vi "Sender.vi"() -> ()   [LabVIEW 2020, in "Data Communication Transmitter.lvlib"]
doc: "Sender VI. Sends the data to the receiver based on the user's inputs."
uses:
  Data Communication Transmitter.lvlib
  Typedefs/Mode Cluster.ctl
  Typedefs/Communication_Mode.ctl
  Typedefs/Communication_Type.ctl
  Typedefs/Medium.ctl
  Typedefs/Data Cluster.ctl
  Typedefs/Sender_Data_Cluster.ctl
  Typedefs/Timing Data.ctl
  Typedefs/Queue Operation_Sender.ctl
  Typedefs/User_Event_Operation.ctl
  Receiver/Typedefs/User event Operations.ctl
  Typedefs/Message type data.ctl
  Classes/Communication/Communication.lvclass
  Typedefs/User_Event_STOP.ctl
  Receiver/Data Communication Receiver.lvlib
  Classes/Children/Intra-Application/Children/Without data/Without Data.lvclass
panel:
  in  "Create Clone":bool
  in  "DATA":T1
  out "error out":errorcluster
  in  "error in":errorcluster
  in  "STOP":bool
  in  "Send":bool
  out "Status indicators":T2
  in  "Medium":T3
  in  "Mode":T4
  # "SENDER"
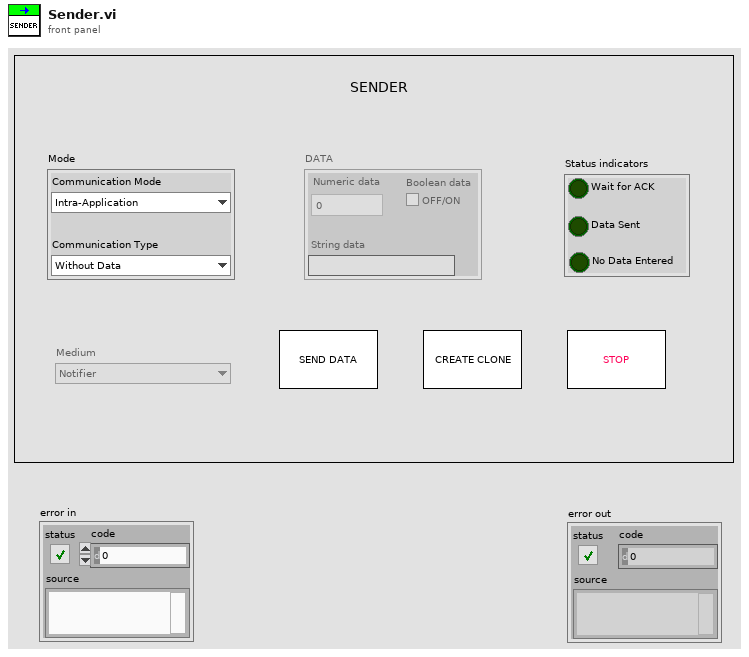
[diagram p1: front panel]
types:
  T1 = typedef "Data Communication Transmitter.lvlib/Data Cluster.ctl" = cluster{"Numeric data":dbl, "String data":string, "Boolean data":bool}
  T2 = cluster{"Wait for ACK":bool, "Data Sent":bool, "No Data Entered":bool}
  T3 = typedef "Data Communication Transmitter.lvlib/Medium.ctl" = enum16{"Notifier", "Queue"}
  T4 = typedef "Data Communication Transmitter.lvlib/Mode Cluster.ctl" = cluster{"Communication Mode":T5, "Communication Type":T6}
  T5 = typedef "Data Communication Transmitter.lvlib/Communication_Mode.ctl" = enum16{"Intra-Application", "Inter-Application"}
  T6 = typedef "Data Communication Transmitter.lvlib/Communication_Type.ctl" = enum16{"Without Data", "With Data"}
  T7 = typedef "Data Communication Transmitter.lvlib/User_Event_Operation.ctl" = enum16{"Create", "Generate", "Destroy", "Get Ref"}
  T8 = typedef "Data Communication Transmitter.lvlib/User event Operations.ctl" = enum16{"Create", "Generate", "Get Ref", "destroy"}
  T9 = typedef "Data Communication Transmitter.lvlib/Queue Operation_Sender.ctl" = enum16{"Create", "Enqueue", "Enstack", "Dequeue", "Flush", "Release"}
  T10 = typedef "Data Communication Transmitter.lvlib/Sender_Data_Cluster.ctl" = cluster{"Enable Controls ref":refnum<vi>[], "Disable Controls ref":refnum<vi>[], "File Path":path, "Status indicators":cluster{"Receiver Offline":bool, "Data Sent":bool, "No Data Entered":bool}, "Medium":T3, "DATA":T1, "Mode Cluster":T4, "Data type":string, "Timing":T11}
  T11 = typedef "Data Communication Transmitter.lvlib/Timing Data.ctl" = cluster{"Start Time":dbl, "Elapsed Time":dbl, "Previous Time":dbl, "Started?":bool, "Paused":bool, "Set Time":dbl}
  T12 = cluster{"Enable Controls ref":refnum<vi>[], "Disable Controls ref":refnum<vi>[]}
  T13 = cluster{"Receiver Offline":bool, "Data Sent":bool, "No Data Entered":bool}
  T14 = enum8{"Enabled", "Disabled", "Disabled and Grayed Out"}
  T15 = typedef "Data Communication Transmitter.lvlib/Message type data.ctl" = cluster{"Message type":string}
  T16 = cluster{"Numeric data":dbl, "String data":string, "Boolean data":bool}
  T17 = typedef "Data Communication Transmitter.lvlib/User_Event_STOP.ctl" = cluster{"STOP":bool}
  T18 = cluster{"Numeric data":bool, "String data":bool, "Boolean data":bool}
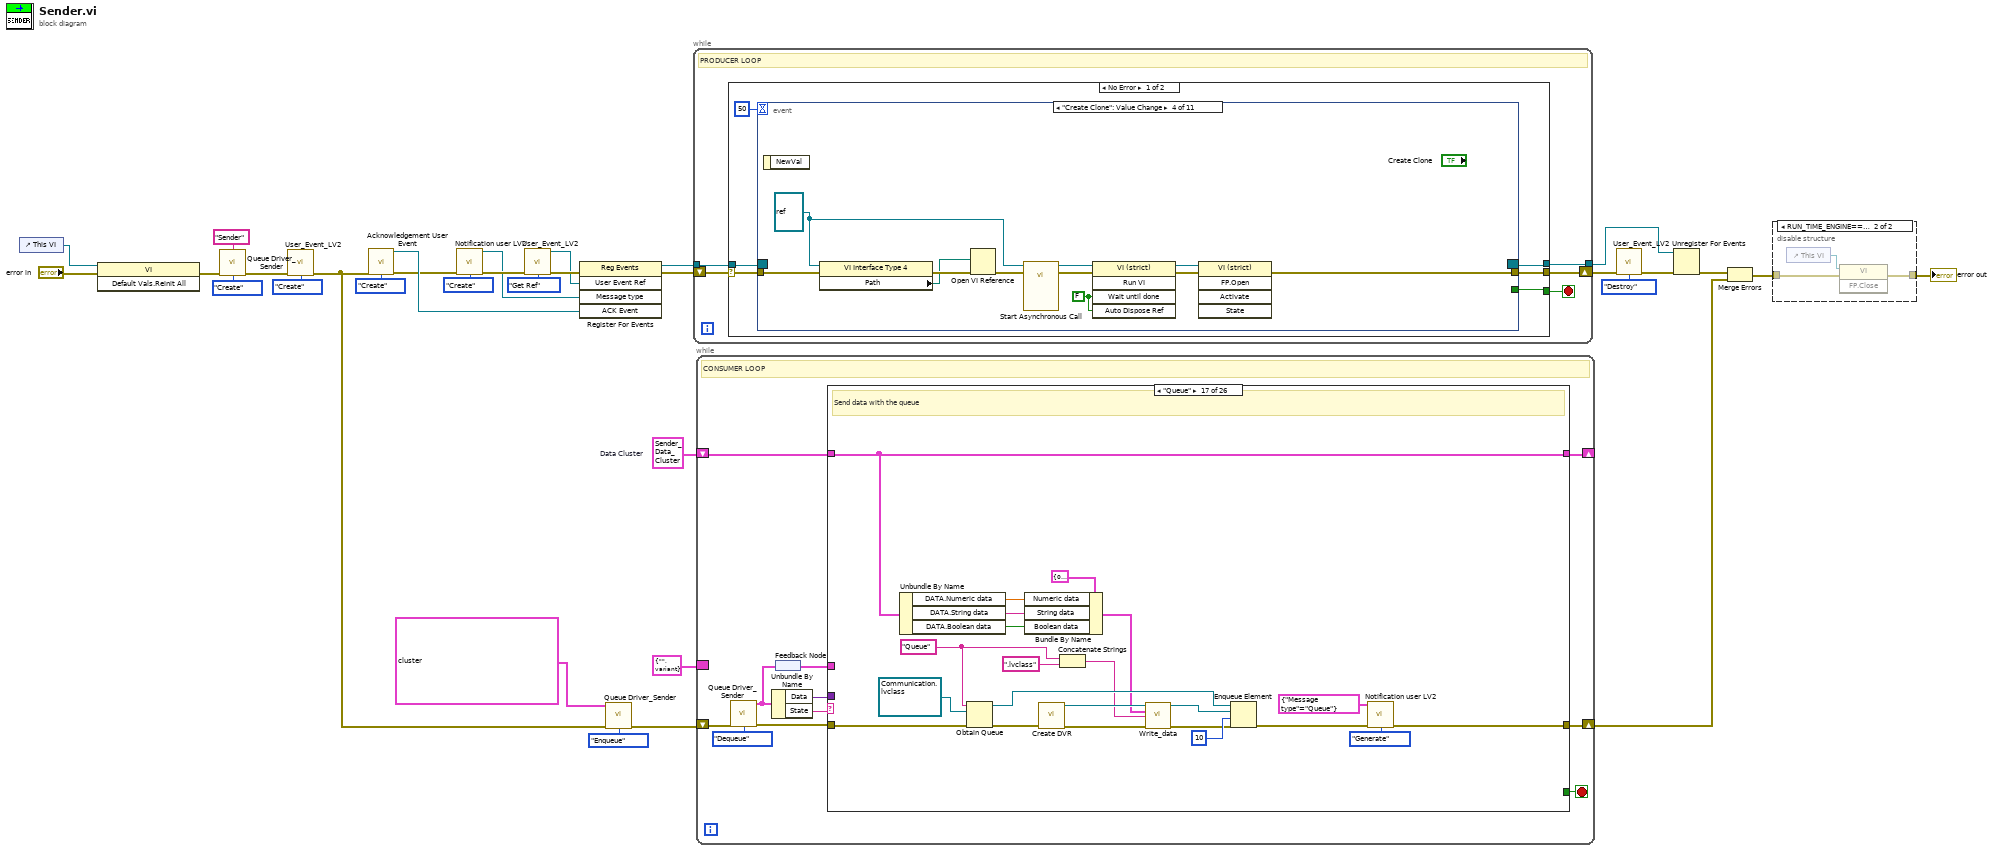
[diagram p0: block diagram]
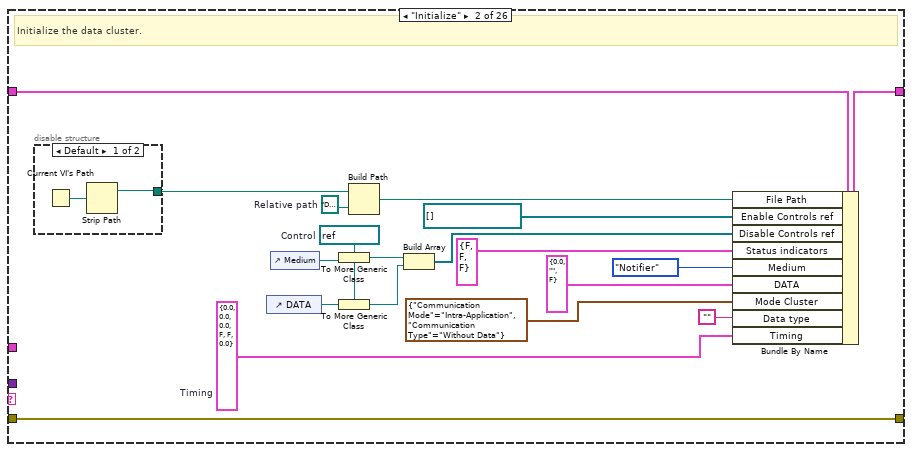
[diagram p4: hidden frame]
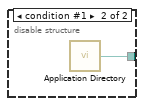
[diagram p5: hidden frame]
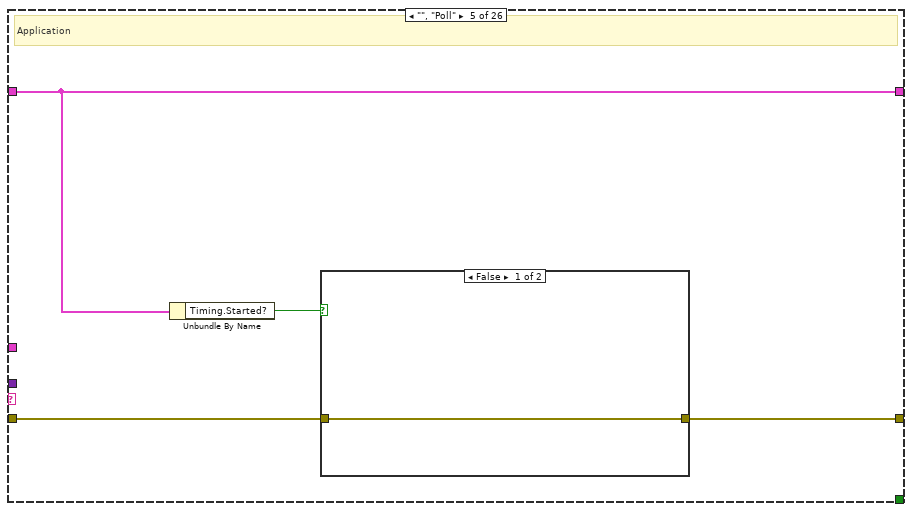
[diagram p8: hidden frame]
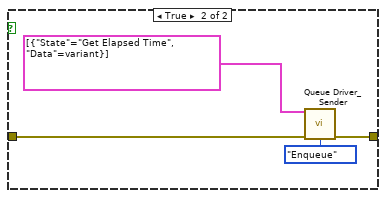
[diagram p9: hidden frame]
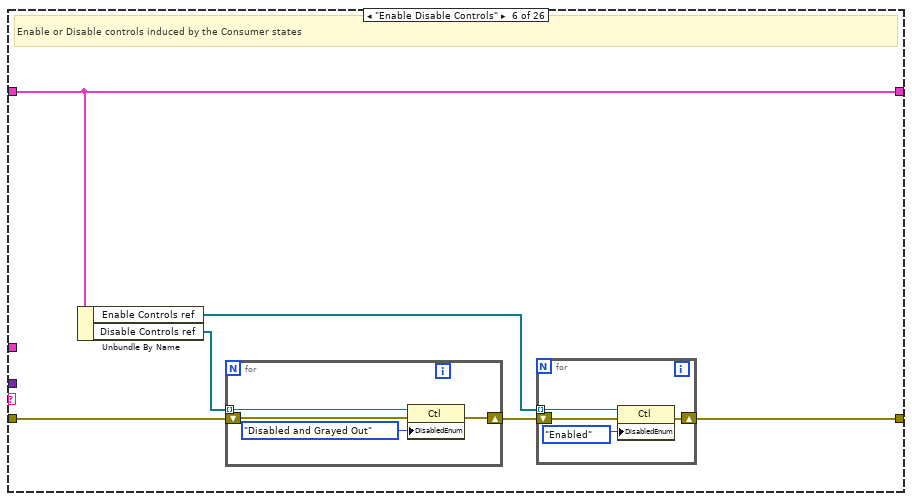
[diagram p10: hidden frame]
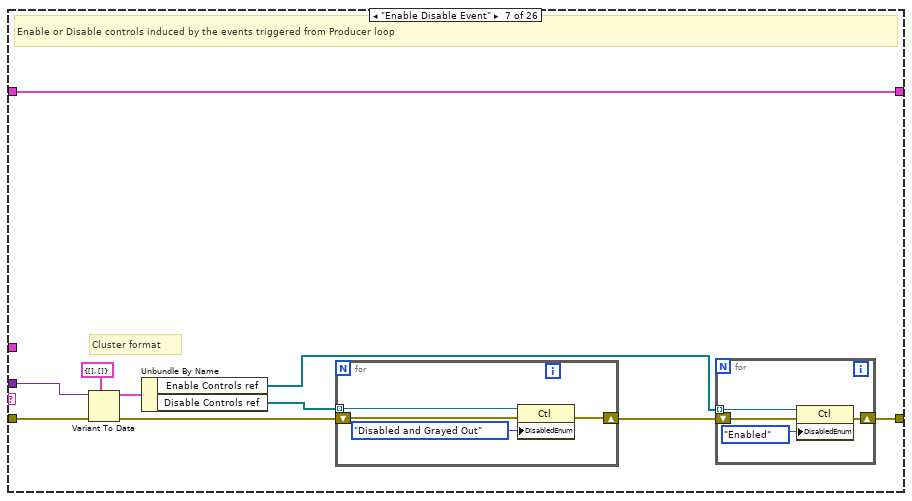
[diagram p11: hidden frame]
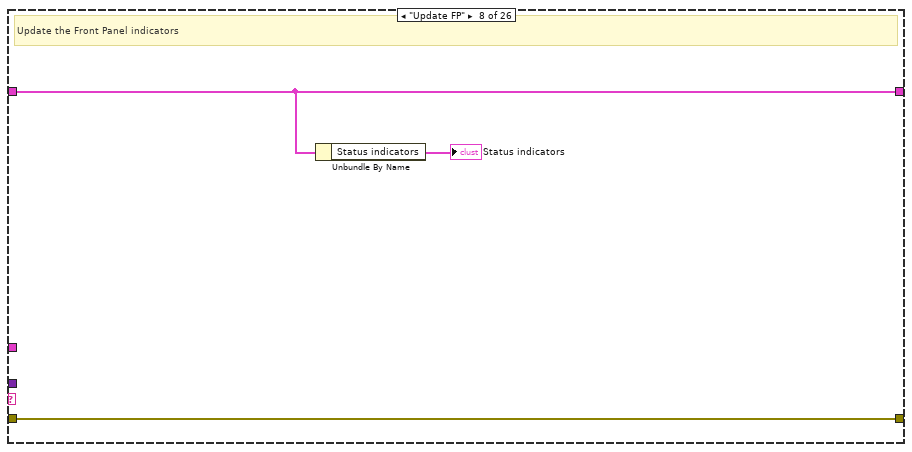
[diagram p12: hidden frame]
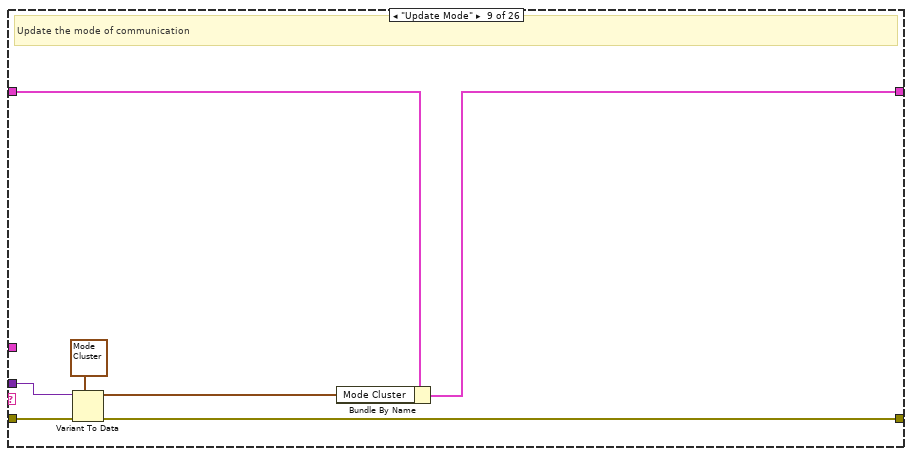
[diagram p13: hidden frame]
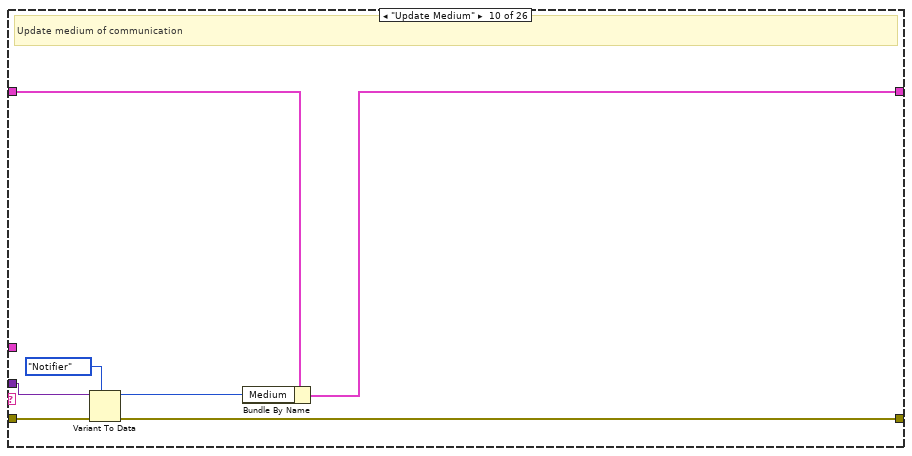
[diagram p14: hidden frame]
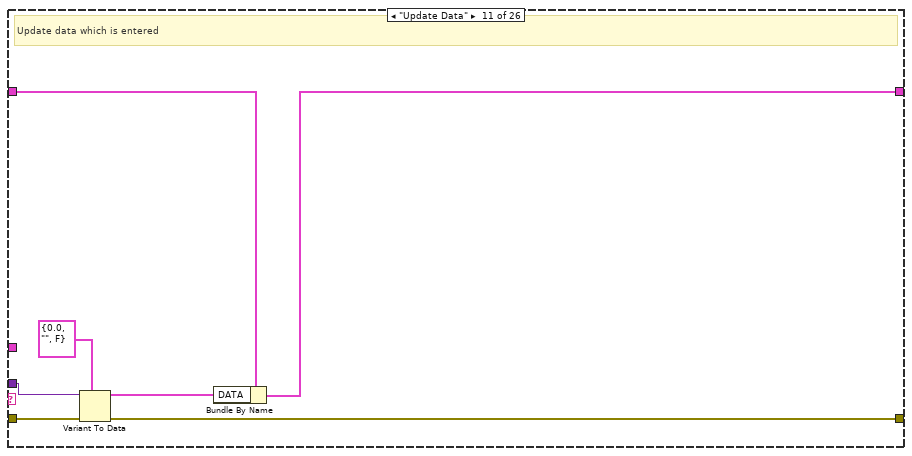
[diagram p15: hidden frame]
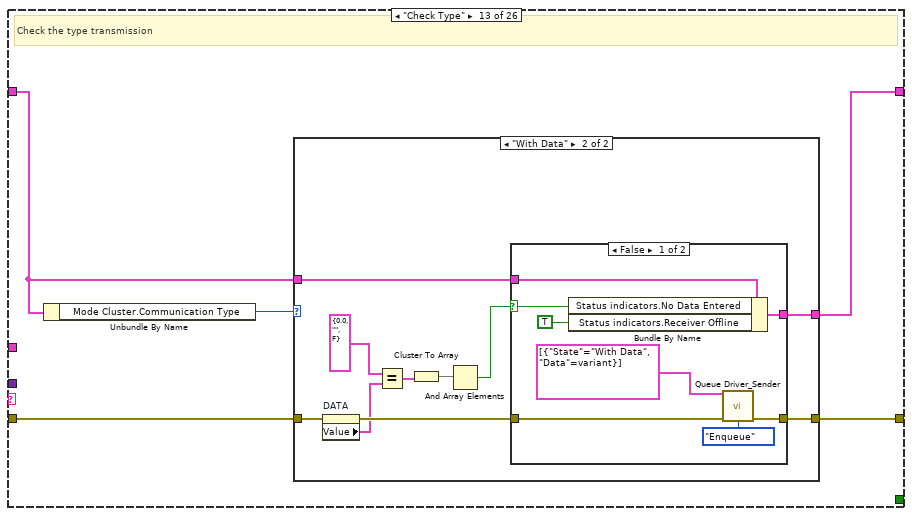
[diagram p17: hidden frame]
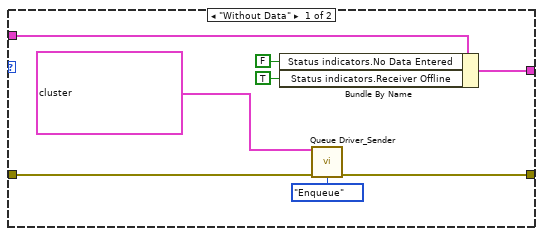
[diagram p18: hidden frame]
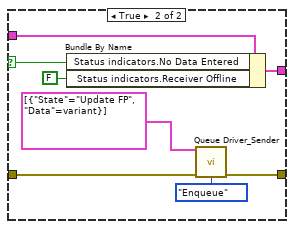
[diagram p19: hidden frame]
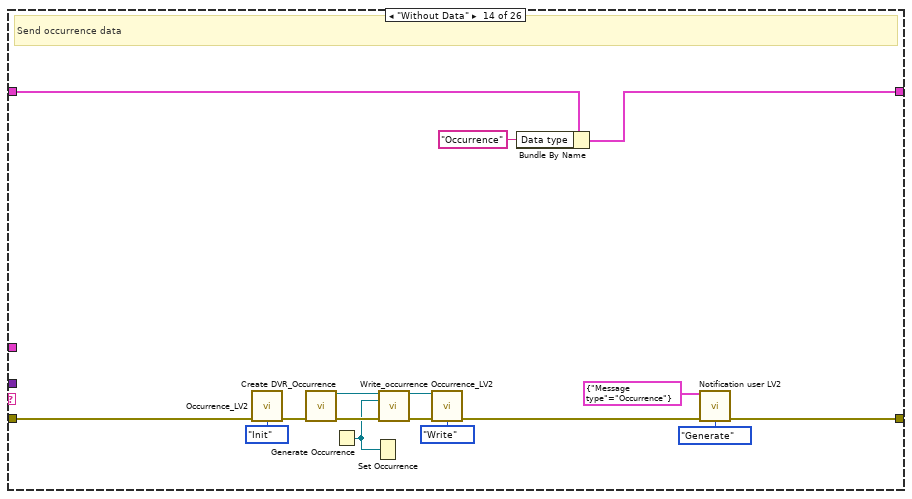
[diagram p20: hidden frame]
diagram:
  w32 = T10 {"Enable Controls ref"=[], "Disable Controls ref"=[], "File Path"=path "", "Status indicators"={"Receiver Offline"=FALSE, "Data Sent"=FALSE, "No Data Entered"=FALSE}, "Medium"=enum."Notifier", "DATA"={"Numeric data"=0.0, "String data"="", "Boolean data"=FALSE}, "Mode Cluster"={"Communication Mode"=enum."Intra-Application", "Communication Type"=enum."Without Data"}, "Data type"="", "Timing"={"Start Time"=0.0, "Elapsed Time"=0.0, "Previous Time"=0.0, "Started?"=FALSE, "Paused"=FALSE, "Set Time"=0.0}}  # Data Cluster
  n1 = control-ref of="This VI"() -> (w8:refnum<vi>)
  n2 = invoke on="Invoke Node" class="VI" method="Default Vals.Reinit All"(reference=w8, error in="error in") -> (error out=w10:errorcluster)  [unwired: 1 in, 2 out]
  n3 = call "Queue Driver_Sender.vi"("Queue Name"="Sender", "Error In"=w10, "Operation"=Queue_Operation_Sender."Create") -> ("Error Out"=w24:errorcluster)  [unwired: 11 in, 1 out]
  n4 = call "User_Event_LV2.vi"("Error In"=w24, "Operation"=User_Event_Operation."Create") -> ("Error Out"=w12:errorcluster)  [unwired: 12 in, 1 out]
  n5 = call "Acknowledgement User Event.vi"("Error in"=w12, "Operations"=User_event_Operations."Create") -> ("ACK Event"=w11:refnum<user-event>, "Error out"=w5:errorcluster)  [unwired: 12 in]
  n6 = call "Notification user LV2.vi"("Error In"=w5, "Operation"=User_Event_Operation."Create") -> ("Message type"=w3:refnum<user-event>, "Error Out"=w4:errorcluster)  [unwired: 12 in]
  n7 = call "User_Event_LV2.vi"("Error In"=w4, "Operation"=User_Event_Operation."Get Ref") -> ("User Event Ref"=w19:refnum<user-event>, "Error Out"=w21:errorcluster)  [unwired: 12 in]
  n8 = register-events(error in=w21, w19, w3, w11) -> (reference out=w18:refnum<event-registration>, error out=w20:errorcluster)  [unwired: 1 in]
  n9 = call "Queue Driver_Sender.vi"("Array of States"=cluster{"State":string, "Data":variant}[] [{"State"="Initialize", "Data"=variant}, {"State"="Enable Disable Controls", "Data"=variant}, {"State"="Update FP", "Data"=variant}], "Error In"=w12, "Operation"=Queue_Operation_Sender."Enqueue") -> ("Error Out"=w27:errorcluster)  [unwired: 11 in, 1 out]
  n10 = while {
    shift-right: [w36] -> w16
    shift-left: w20 -> [w37]
    tunnel: w18 -> [w35]
    tunnel: [w33] -> w13
    stop <- w34 stop-if-true
    # "PRODUCER LOOP"
    n11 = case shown="No Error" w37 {
      selector: w37 -> [w43 w158]
      tunnel: [w42 w164] -> w36
      tunnel: w35 -> [w41 w156]
      tunnel: [w40 _] -> w34
      tunnel: [w39 w156] -> w33
      frame No Error {
        n12 = event shown="[3] \"Create Clone\": Value Change" {
          selector: w41 -> [_ w46 _ _ _ _ _ _ _ _ _]
          dyn-events: [_ w46 _ _ _ _ _ _ _ _ _] -> w39
          timeout: 50 -> [_ _ _ _ _ _ _ _ _ _ _]
          tunnel: w43 -> [w45 w47 w52 w64 w71 w79 w89 w98 w107 w113 w118]
          tunnel: [w45 w47 w50 w55 w70 w78 w88 w103 w108 w114 w117] -> w42
          tunnel: [FALSE ("STOP") w48 FALSE ("STOP") _ FALSE ("STOP") FALSE ("STOP") FALSE ("STOP") FALSE ("STOP") FALSE ("STOP") FALSE ("STOP") FALSE ("STOP")] -> w40
          event Timeout {
            n13 = event-data() -> ()  [unwired: 1 in, 1 out]
          }
          event User Event {
            # "Consumer Stop Event"
            n14 = event-data() -> ("STOP"=w48:bool)  [unwired: 1 in]
          }
          event "Send": Value Change {
            # "Send Data"
            n15 = event-data() -> ()  [unwired: 1 in, 1 out]
            n16 = call "Queue Driver_Sender.vi"("Array of States"=cluster{"State":string, "Data":variant}[] [{"State"="Check Type", "Data"=variant}], "Error In"=w52, "Operation"=Queue_Operation_Sender."Enqueue") -> ("Error Out"=w50:errorcluster)  [unwired: 11 in, 1 out]
          }
          event "Create Clone": Value Change {
            w56 = FALSE ("Wait Until Done")
            w59 = refnum<vi> refnum
            n17 = event-data() -> ()  [unwired: 1 in, 1 out]
            n18 = property class="VI Interface Type 4"(reference=w59, error in=w64) -> (error out=w63:errorcluster, "Path"=w61:path)  [unwired: 1 out]
            n19 = Open VI Reference(vi path=w61, error in (no error)=w63) -> (error out=w62:errorcluster)  [unwired: 4 in, 1 out]
            n20 = call-by-ref "Start Asynchronous Call"(reference=w59, error in=w62) -> (reference out=w57:refnum<vi>, error out=w60:errorcluster)  [unwired: 15 in, 1 out]
            n21 = invoke class="VI (strict)" method="Run VI"(reference=w57, error in=w60, "Wait until done"=w56, "Auto Dispose Ref"=w56) -> (reference out=w54:refnum<vi>, error out=w58:errorcluster)  [unwired: 1 in, 3 out]
            n22 = invoke class="VI (strict)" method="FP.Open"(reference=w54, error in=w58) -> (error out=w55:errorcluster)  [unwired: 3 in, 4 out]
          }
          event Value Change {
            # "Update mode to cluster"
            n23 = event-data() -> ("NewVal"=w65:T4)  [unwired: 1 in]
            n24 = To Variant(anything=w65) -> (Variant=w66:variant)
            n25 = Bundle By Name(cluster=cluster{"State":string, "Data":variant} {"State"="", "Data"=variant} ("Data Cluster"), "State"="Update Mode", "Data"=w66) -> (w73:cluster{"State":string, "Data":variant})
            n26 = Build Array(w73) -> (w69:cluster{"State":string, "Data":variant}[])
            n27 = call "Queue Driver_Sender.vi"("Array of States"=w69, "Error In"=w71, "Operation"=Queue_Operation_Sender."Enqueue") -> ("Error Out"=w70:errorcluster)  [unwired: 11 in, 1 out]
          }
          event Value Change {
            # "Update medium of data transmission"
            n28 = event-data() -> ("NewVal"=w75:T3)  [unwired: 1 in]
            n29 = To Variant(anything=w75) -> (Variant=w76:variant)
            n30 = Bundle By Name(cluster=cluster{"State":string, "Data":variant} {"State"="", "Data"=variant} ("Data Cluster"), "State"="Update Medium", "Data"=w76) -> (w82:cluster{"State":string, "Data":variant})
            n31 = Build Array(w82) -> (w80:cluster{"State":string, "Data":variant}[])
            n32 = call "Queue Driver_Sender.vi"("Array of States"=w80, "Error In"=w79, "Operation"=Queue_Operation_Sender."Enqueue") -> ("Error Out"=w78:errorcluster)  [unwired: 11 in, 1 out]
          }
          event Value Change {
            # "Update change in input data"
            n33 = event-data() -> ("NewVal"=w85:T1)  [unwired: 1 in]
            n34 = To Variant(anything=w85) -> (Variant=w86:variant)
            n35 = Bundle By Name(cluster=cluster{"State":string, "Data":variant} {"State"="", "Data"=variant} ("Data Cluster"), "State"="Update Data", "Data"=w86) -> (w92:cluster{"State":string, "Data":variant})
            n36 = Build Array(w92) -> (w90:cluster{"State":string, "Data":variant}[])
            n37 = call "Queue Driver_Sender.vi"("Array of States"=w90, "Error In"=w89, "Operation"=Queue_Operation_Sender."Enqueue") -> ("Error Out"=w88:errorcluster)  [unwired: 11 in, 1 out]
          }
          event User Event {
            # "Acknowledgemnt from the receiver"
            n38 = event-data() -> ()  [unwired: 1 in, 1 out]
            n39 = property on="Data Sent" class="Bool (strict)"(error in=w98, "Value"=TRUE) -> (error out=w99:errorcluster)  [unwired: 1 in, 1 out]
            n40 = Bundle By Name(cluster=cluster{"State":string, "Data":variant} {"State"="", "Data"=variant} ("input cluster"), "State"="Start Timer") -> (w101:cluster{"State":string, "Data":variant})
            n41 = Build Array(w101) -> (w100:cluster{"State":string, "Data":variant}[])
            n42 = call "Queue Driver_Sender.vi"("Array of States"=w100, "Error In"=w99, "Operation"=Queue_Operation_Sender."Enqueue") -> ("Error Out"=w103:errorcluster)  [unwired: 11 in, 1 out]
          }
          event Panel Close? {
            # "Handling panel close"
            n43 = event-data() -> ()  [unwired: 1 in, 1 out]
            n44 = call "Queue Driver_Sender.vi"("Array of States"=cluster{"State":string, "Data":variant}[] [{"State"="Exit", "Data"=variant}], "Error In"=w107, "Operation"=Queue_Operation_Sender."Enqueue") -> ("Error Out"=w108:errorcluster)  [unwired: 11 in, 1 out]
            n45 = event-data ("Event Filter Node")("Discard?"=TRUE) -> ()  [unwired: 1 in, 1 out]
          }
          event "STOP": Value Change {
            # "Handle terminate with stop"
            n46 = event-data() -> ()  [unwired: 1 in, 1 out]
            n47 = call "Queue Driver_Sender.vi"("Array of States"=cluster{"State":string, "Data":variant}[] [{"State"="Exit", "Data"=variant}], "Error In"=w113, "Operation"=Queue_Operation_Sender."Enqueue") -> ("Error Out"=w114:errorcluster)  [unwired: 11 in, 1 out]
          }
          event Value Change {
            # "Enable and disbale controls"
            n48 = event-data() -> ("NewVal"=w119:T6)  [unwired: 1 in]
            n49 = case shown="\"Without Data\"" w119 {
              tunnel: w118 -> [w120 w138]
              tunnel: [w128 w147] -> w117
              frame "With Data" {
                w123 = refnum<vi> refnum  # Control
                n50 = control-ref of="DATA"() -> (w122:refnum<vi>)
                n51 = control-ref of="Medium"() -> (w136:refnum<vi>)
                n52 = To More Generic Class(target class=w123, reference=w136) -> (generic class reference=w135:refnum<vi>)
                n53 = To More Generic Class(target class=w123, reference=w122) -> (generic class reference=w121:refnum<vi>)
                n54 = Build Array(w135, w121) -> (w126:refnum<vi>[])
                n55 = Bundle By Name(cluster=T12 {"Enable Controls ref"=[], "Disable Controls ref"=[]} ("input cluster"), "Disable Controls ref"=refnum<vi>[] [], "Enable Controls ref"=w126) -> (w125:T12)
                n56 = To Variant(anything=w125) -> (Variant=w133:variant)
                n57 = Bundle By Name(cluster=cluster{"State":string, "Data":variant} {"State"="", "Data"=variant} ("Data Cluster"), "State"="Enable Disable Event", "Data"=w133) -> (w131:cluster{"State":string, "Data":variant})
                n58 = Build Array(w131) -> (w129:cluster{"State":string, "Data":variant}[])
                n59 = call "Queue Driver_Sender.vi"("Array of States"=w129, "Error In"=w120, "Operation"=Queue_Operation_Sender."Enqueue") -> ("Error Out"=w128:errorcluster)  [unwired: 11 in, 1 out]
              }
              frame "Without Data" {
                w142 = refnum<vi> refnum  # Control
                n60 = control-ref of="DATA"() -> (w141:refnum<vi>)
                n61 = control-ref of="Medium"() -> (w155:refnum<vi>)
                n62 = To More Generic Class(target class=w142, reference=w155) -> (generic class reference=w154:refnum<vi>)
                n63 = To More Generic Class(target class=w142, reference=w141) -> (generic class reference=w140:refnum<vi>)
                n64 = Build Array(w154, w140) -> (w145:refnum<vi>[])
                n65 = Bundle By Name(cluster=T12 {"Enable Controls ref"=[], "Disable Controls ref"=[]} ("input cluster"), "Enable Controls ref"=refnum<vi>[] [] ("Disable Controls ref"), "Disable Controls ref"=w145) -> (w144:T12)
                n66 = property on="No Data Entered" class="Bool (strict)"(error in=w138, "Value"=FALSE) -> (error out=w139:errorcluster)  [unwired: 1 in, 1 out]
                n67 = To Variant(anything=w144) -> (Variant=w152:variant)
                n68 = Bundle By Name(cluster=cluster{"State":string, "Data":variant} {"State"="", "Data"=variant} ("Data Cluster"), "State"="Enable Disable Event", "Data"=w152) -> (w150:cluster{"State":string, "Data":variant})
                n69 = Build Array(w150) -> (w148:cluster{"State":string, "Data":variant}[])
                n70 = call "Queue Driver_Sender.vi"("Array of States"=w148, "Error In"=w139, "Operation"=Queue_Operation_Sender."Enqueue") -> ("Error Out"=w147:errorcluster)  [unwired: 11 in, 1 out]
              }
            }
          }
        }
      }
      frame Error {
        n71 = To Variant(anything=w158) -> (Variant=w161:variant)
        n72 = call <vilib>:"Clear Errors.vi"("error in (no error)"=w158) -> ("error out"=w157:errorcluster)  [unwired: 5 in, 1 out]
        n73 = Bundle By Name(cluster=cluster{"State":string, "Data":variant} {"State"="", "Data"=variant} ("Data Cluster"), "State"="Producer Error", "Data"=w161) -> (w160:cluster{"State":string, "Data":variant})
        n74 = Build Array(w160) -> (w159:cluster{"State":string, "Data":variant}[])
        n75 = call "Queue Driver_Sender.vi"("Array of States"=w159, "Error In"=w157, "Operation"=Queue_Operation_Sender."Enqueue") -> ("Error Out"=w164:errorcluster)  [unwired: 11 in, 1 out]
      }
    }
  }
  n76 = while {
    shift-right: [w176] -> w26
    shift-left: w27 -> [w168]
    shift-right: [w172] -> _
    shift-left: w32 -> [w173]
    border: cluster{"State":string, "Data":variant} {"State"="", "Data"=variant} ("Data Cluster") -> [_]
    stop <- w174 stop-if-true
    # "CONSUMER LOOP"
    n77 = call "Queue Driver_Sender.vi"("Error In"=w168, "Operation"=Queue_Operation_Sender."Dequeue") -> ("Data Cluster"=w166:cluster{"State":string, "Data":variant}, "Error Out"=w169:errorcluster)  [unwired: 12 in]
    n78 = Unbundle By Name(w166) -> ("Data"=w175:variant, "State"=w171:string)
    n79 = feedback #1() -> (w170:cluster{"State":string, "Data":variant})
    n80 = feedback-in #1(w166) -> ()
    n81 = case shown="\"Queue\"" w171 {
      tunnel: [w178 w180 w202 w204 w206 w218 w235 w248 w249 w256 w266 w271 w274 w321 w329 w363 w381 w390 w393 w403 w412 w442 w445 w474 w493 w495] -> w176
      tunnel: w169 -> [w178 w180 w202 w204 w207 w215 w231 w248 w255 w262 w269 w271 w275 w320 w330 w358 w388 w390 w393 w403 w414 w442 w446 w471 w493 w498]
      tunnel: w175 -> [_ _ _ _ _ _ w230 _ w254 w261 w268 _ _ _ _ _ _ _ _ _ _ _ _ w473 _ _]
      tunnel: [_ _ _ _ _ _ _ _ _ _ _ _ _ _ _ _ _ _ _ _ _ _ _ _ _ TRUE] -> w174
      tunnel: w173 -> [w177 w194 w201 w203 w208 w214 w237 w247 w252 w259 w265 w270 w273 w326 w328 w366 w386 w389 w392 w402 w417 w441 w456 w481 w492 w503]
      tunnel: [w177 w193 w201 w203 w208 w214 w237 w247 w250 w258 w264 w270 w272 w325 w327 w366 w386 w389 w391 w401 w418 w441 w456 w481 w492 w503] -> w172
      tunnel: w170 -> [_ _ _ _ _ _ _ _ _ _ _ _ _ _ _ _ _ _ _ _ _ _ w444 _ _ _]
      frame "***Initialize***" {
      }
      frame "Initialize" {
        w181 = T11 {"Start Time"=0.0, "Elapsed Time"=0.0, "Previous Time"=0.0, "Started?"=FALSE, "Paused"=FALSE, "Set Time"=0.0}  # Timing
        w188 = refnum<vi> refnum  # Control
        w196 = path "Data/Accounts.csv"  # Relative path
        # "Initialize the data cluster."
        n82 = disable-structure "Conditional Disable Structure" shown="Default" {
          disable-tunnel: [w199 w200] -> w197
          frame condition #0 (active) {
            n83 = Current VI's Path() -> (path=w198:path)
            n84 = Strip Path(path=w198) -> (stripped path=w199:path)  [unwired: 1 out]
          }
          frame condition #1 {
            n85 = call <vilib>:"Application Directory.vi"() -> ("Application Directory"=w200:path)
          }
        }
        n86 = control-ref of="DATA"() -> (w187:refnum<vi>)
        n87 = control-ref of="Medium"() -> (w191:refnum<vi>)
        n88 = To More Generic Class(target class=w188, reference=w191) -> (generic class reference=w190:refnum<vi>)
        n89 = To More Generic Class(target class=w188, reference=w187) -> (generic class reference=w186:refnum<vi>)
        n90 = Build Path(base path=w197, name or relative path=w196) -> (appended path=w195:path)
        n91 = Build Array(w190, w186) -> (w189:refnum<vi>[])
        n92 = Bundle By Name(cluster=w194, "File Path"=w195, "Enable Controls ref"=refnum<vi>[] [], "Disable Controls ref"=w189, "Status indicators"=T13 {"Receiver Offline"=FALSE, "Data Sent"=FALSE, "No Data Entered"=FALSE}, "Medium"=Medium."Notifier", "DATA"=T1 {"Numeric data"=0.0, "String data"="", "Boolean data"=FALSE}, "Mode Cluster"=T4 {"Communication Mode"=enum."Intra-Application", "Communication Type"=enum."Without Data"}, "Data type"="" ("Empty String Constant"), "Timing"=w181) -> (w193:T10)
      }
      frame "***FP Related***" {
      }
      frame Default {
      }
      frame "", "Poll" {
        # "Application"
        n93 = Unbundle By Name(w208) -> ("Timing.Started?"=w205:bool)
        n94 = case shown="False" w205 {
          tunnel: w207 -> [w209 w212]
          tunnel: [w209 w211] -> w206
          frame False {
          }
          frame True {
            n95 = call "Queue Driver_Sender.vi"("Array of States"=cluster{"State":string, "Data":variant}[] [{"State"="Get Elapsed Time", "Data"=variant}], "Error In"=w212, "Operation"=Queue_Operation_Sender."Enqueue") -> ("Error Out"=w211:errorcluster)  [unwired: 11 in, 1 out]
          }
        }
      }
      frame "Enable Disable Controls" {
        # "Enable or Disable controls induced by the Consumer states"
        n96 = Unbundle By Name(w214) -> ("Enable Controls ref"=w217:refnum<vi>[], "Disable Controls ref"=w216:refnum<vi>[])
        n97 = for {
          tunnel: w216 -> [w224] mode=indexing
          shift-right: [w225] -> w219
          shift-left: w215 -> [w227]
          n98 = property on="Property Node" class="Ctl"(reference=w224, error in=w227, "DisabledEnum"=T14."Disabled and Grayed Out" ("Disabled")) -> (error out=w225:errorcluster)  [unwired: 1 out]
        }
        n99 = for {
          shift-right: [w221] -> w218
          shift-left: w219 -> [w222]
          tunnel: w217 -> [w220] mode=indexing
          n100 = property on="Property Node" class="Ctl"(reference=w220, error in=w222, "DisabledEnum"=T14."Enabled" ("Disabled")) -> (error out=w221:errorcluster)  [unwired: 1 out]
        }
      }
      frame "Enable Disable Event" {
        # "Cluster format"
        # "Enable or Disable controls induced by the events triggered from Producer loop"
        n101 = Variant To Data(error in=w231, type=T12 {"Enable Controls ref"=[], "Disable Controls ref"=[]} ("input cluster"), Variant=w230) -> (data=w233:T12, error out=w232:errorcluster)
        n102 = Unbundle By Name(w233) -> ("Enable Controls ref"=w228:refnum<vi>[], "Disable Controls ref"=w229:refnum<vi>[])
        n103 = for {
          shift-right: [w243] -> w236
          shift-left: w232 -> [w245]
          tunnel: w229 -> [w242] mode=indexing
          n104 = property on="Property Node" class="Ctl"(reference=w242, error in=w245, "DisabledEnum"=T14."Disabled and Grayed Out" ("Disabled")) -> (error out=w243:errorcluster)  [unwired: 1 out]
        }
        n105 = for {
          shift-right: [w239] -> w235
          shift-left: w236 -> [w240]
          tunnel: w228 -> [w238] mode=indexing
          n106 = property on="Property Node" class="Ctl"(reference=w238, error in=w240, "DisabledEnum"=T14."Enabled" ("Disabled")) -> (error out=w239:errorcluster)  [unwired: 1 out]
        }
      }
      frame "Update FP" {
        # "Update the Front Panel indicators"
        n107 = Unbundle By Name(w247) -> ("Status indicators"=→"Status indicators":T13)
      }
      frame "Update Mode" {
        # "Update the mode of communication"
        n108 = Variant To Data(error in=w255, type=T4 {"Communication Mode"=enum."Intra-Application", "Communication Type"=enum."Without Data"} ("Mode Cluster"), Variant=w254) -> (data=w251:T4, error out=w249:errorcluster)
        n109 = Bundle By Name(cluster=w252, "Mode Cluster"=w251) -> (w250:T10)
      }
      frame "Update Medium" {
        # "Update medium of communication"
        n110 = Variant To Data(error in=w262, type=Medium."Notifier" ("Medium"), Variant=w261) -> (data=w257:T3, error out=w256:errorcluster)
        n111 = Bundle By Name(cluster=w259, "Medium"=w257) -> (w258:T10)
      }
      frame "Update Data" {
        # "Update data which is entered"
        n112 = Variant To Data(error in=w269, type=T1 {"Numeric data"=0.0, "String data"="", "Boolean data"=FALSE} ("DATA"), Variant=w268) -> (data=w263:T1, error out=w266:errorcluster)
        n113 = Bundle By Name(cluster=w265, "DATA"=w263) -> (w264:T10)
      }
      frame "***Operations***" {
      }
      frame "Check Type" {
        # "Check the type transmission"
        n114 = Unbundle By Name(w273) -> ("Mode Cluster.Communication Type"=w276:T6)
        n115 = case shown="\"With Data\"" w276 {
          tunnel: w275 -> [w283 w292]
          tunnel: [w282 w294] -> w274
          tunnel: w273 -> [w280 w287]
          tunnel: [w278 w286] -> w272
          frame "Without Data" {
            n116 = Bundle By Name(cluster=w280, "Status indicators.No Data Entered"=FALSE, "Status indicators.Receiver Offline"=TRUE) -> (w278:T10)
            n117 = call "Queue Driver_Sender.vi"("Array of States"=cluster{"State":string, "Data":variant}[] [{"State"="Without Data", "Data"=variant}, {"State"="Update FP", "Data"=variant}], "Error In"=w283, "Operation"=Queue_Operation_Sender."Enqueue") -> ("Error Out"=w282:errorcluster)  [unwired: 11 in, 1 out]
          }
          frame "With Data" {
            n118 = property on="DATA" class="Clust (strict)"(error in=w292) -> (error out=w293:errorcluster, "Value"=w290:T1)  [unwired: 1 in, 1 out]
            n119 = Equal?(x=T1 {"Numeric data"=0.0, "String data"="", "Boolean data"=FALSE} ("DATA"), y=w290) -> (x = y?=w289:T18)
            n120 = Cluster To Array(cluster=w289) -> (array=w288:bool[])
            n121 = And Array Elements(Boolean array=w288) -> (logical AND=w285:bool)
            n122 = case shown="False" w285 {
              selector: w285 -> [w297 w309]
              tunnel: [w301 w304] -> w294
              tunnel: w293 -> [w299 w305]
              tunnel: w287 -> [w298 w310]
              tunnel: [w296 w308] -> w286
              frame False {
                n123 = Bundle By Name(cluster=w298, "Status indicators.No Data Entered"=w297, "Status indicators.Receiver Offline"=TRUE) -> (w296:T10)
                n124 = call "Queue Driver_Sender.vi"("Array of States"=cluster{"State":string, "Data":variant}[] [{"State"="With Data", "Data"=variant}], "Error In"=w299, "Operation"=Queue_Operation_Sender."Enqueue") -> ("Error Out"=w301:errorcluster)  [unwired: 11 in, 1 out]
              }
              frame True {
                n125 = Bundle By Name(cluster=w310, "Status indicators.No Data Entered"=w309, "Status indicators.Receiver Offline"=FALSE) -> (w308:T10)
                n126 = call "Queue Driver_Sender.vi"("Array of States"=cluster{"State":string, "Data":variant}[] [{"State"="Update FP", "Data"=variant}], "Error In"=w305, "Operation"=Queue_Operation_Sender."Enqueue") -> ("Error Out"=w304:errorcluster)  [unwired: 11 in, 1 out]
              }
            }
          }
        }
      }
      frame "Without Data" {
        # "Send occurrence data"
        n127 = call "Occurrence_LV2.vi"("Error In"=w320, "Operation"=enum16{"Init", "Read", "Write"}."Init") -> ("Error Out"=w319:errorcluster)  [unwired: 12 in, 1 out]
        n128 = call "Create DVR_Occurrence.vi"("error in (no error)"=w319) -> ("Without data DVR reference"=w317:refnum<data-value>, "error out"=w318:errorcluster)  [unwired: 13 in]
        n129 = Generate Occurrence() -> (w311:refnum<k4>)
        n130 = Set Occurrence(w311) -> ()
        n131 = call "Write_occurrence.vi"("Without data DVR reference in"=w317, "Occurrence Ref"=w311, "error in (no error)"=w318) -> ("Without data DVR reference out"=w313:refnum<data-value>, "error out"=w314:errorcluster)  [unwired: 11 in]
        n132 = call "Occurrence_LV2.vi"("Without data DVR reference in"=w313, "Error In"=w314, "Operation"=enum16{"Init", "Read", "Write"}."Write") -> ("Error Out"=w312:errorcluster)  [unwired: 11 in, 1 out]
        n133 = Bundle By Name(cluster=w326, "Data type"="Occurrence") -> (w325:T10)
        n134 = call "Notification user LV2.vi"("Data"=T15 {"Message type"="Occurrence"}, "Error In"=w312, "Operation"=User_Event_Operation."Generate") -> ("Error Out"=w321:errorcluster)  [unwired: 11 in, 1 out]
      }
      frame "With Data" {
        # "Choose wheather queue or notifier"
        n135 = Unbundle By Name(w328) -> ("Medium"=w331:T3)
        n136 = case shown="\"Notifier\"" w331 {
          tunnel: w330 -> [w336 w343]
          tunnel: [w335 w342] -> w329
          tunnel: w328 -> [w333 w341]
          tunnel: [w332 w339] -> w327
          frame "Notifier" {
            n137 = Bundle By Name(cluster=w333, "Data type"="Notifier") -> (w332:T10)
            n138 = call "Queue Driver_Sender.vi"("Array of States"=cluster{"State":string, "Data":variant}[] [{"State"="Notifier", "Data"=variant}], "Error In"=w336, "Operation"=Queue_Operation_Sender."Enqueue") -> ("Error Out"=w335:errorcluster)  [unwired: 11 in, 1 out]
          }
          frame "Queue" {
            n139 = Bundle By Name(cluster=w341, "Data type"="Queue") -> (w339:T10)
            n140 = call "Queue Driver_Sender.vi"("Array of States"=cluster{"State":string, "Data":variant}[] [{"State"="Queue", "Data"=variant}], "Error In"=w343, "Operation"=Queue_Operation_Sender."Enqueue") -> ("Error Out"=w342:errorcluster)  [unwired: 11 in, 1 out]
          }
        }
      }
      frame "Notifier" {
        w356 = "Notifier" ("name (unnamed)")
        # "Send data with the queue"
        n141 = Unbundle By Name(w366) -> ("DATA.Numeric data"=w361:dbl, "DATA.String data"=w360:string, "DATA.Boolean data"=w359:bool)
        n142 = Obtain Notifier(name (unnamed)=w356, notification data type=refnum<data-value> refnum ("DVR Out"), error in (no error)=w358) -> (notifier out=w346:refnum<notifier>, error out=w354:errorcluster)  [unwired: 1 in, 1 out]
        n143 = Bundle By Name(cluster=T16 {"Numeric data"=0.0, "String data"="", "Boolean data"=FALSE} ("DATA"), "Numeric data"=w361, "String data"=w360, "Boolean data"=w359) -> (w351:T16)
        n144 = call "Create DVR.vi"("error in (no error)"=w354) -> ("DVR Out"=w350:refnum<data-value>, "error out"=w353:errorcluster)  [unwired: 13 in]
        n145 = Concatenate Strings(w356, "s.lvclass" ("string")) -> (w349:string)
        n146 = call "Write_data.vi"("DVR In"=w350, "DATA"=w351, "Name"=w349, "error in"=w353) -> ("DVR Out"=w348:refnum<data-value>, "error out"=w352:errorcluster)  [unwired: 10 in]
        n147 = Send Notification(notification=w348, notifier=w346, error in (no error)=w352) -> (error out=w357:errorcluster)  [unwired: 1 out]
        n148 = call "Notification user LV2.vi"("Data"=T15 {"Message type"="Notifier"}, "Error In"=w357, "Operation"=User_Event_Operation."Generate") -> ("Error Out"=w363:errorcluster)  [unwired: 11 in, 1 out]
      }
      frame "Queue" {
        w376 = "Queue" ("name (unnamed)")
        # "Send data with the queue"
        n149 = Unbundle By Name(w386) -> ("DATA.Numeric data"=w379:dbl, "DATA.String data"=w378:string, "DATA.Boolean data"=w377:bool)
        n150 = Obtain Queue(name (unnamed)=w376, element data type=refnum<data-value> refnum ("DVR Out"), error in (no error)=w388) -> (queue out=w385:refnum<queue>, error out=w373:errorcluster)  [unwired: 2 in, 1 out]
        n151 = Bundle By Name(cluster=T16 {"Numeric data"=0.0, "String data"="", "Boolean data"=FALSE} ("DATA"), "Numeric data"=w379, "String data"=w378, "Boolean data"=w377) -> (w370:T16)
        n152 = call "Create DVR.vi"("error in (no error)"=w373) -> ("DVR Out"=w372:refnum<data-value>, "error out"=w374:errorcluster)  [unwired: 13 in]
        n153 = Concatenate Strings(w376, ".lvclass" ("string")) -> (w371:string)
        n154 = call "Write_data.vi"("DVR In"=w372, "DATA"=w370, "Name"=w371, "error in"=w374) -> ("DVR Out"=w367:refnum<data-value>, "error out"=w369:errorcluster)  [unwired: 10 in]
        n155 = Enqueue Element(queue=w385, element=w367, timeout in ms (-1)=10, error in (no error)=w369) -> (error out=w382:errorcluster)  [unwired: 2 out]
        n156 = call "Notification user LV2.vi"("Data"=T15 {"Message type"="Queue"}, "Error In"=w382, "Operation"=User_Event_Operation."Generate") -> ("Error Out"=w381:errorcluster)  [unwired: 11 in, 1 out]
      }
      frame "/***Timing***/" {
      }
      frame "Start Timer" {
        # "Start timer"
        n157 = in-place "In Place Element Structure" {
          w396 = 0.0 ("Timing.Previous Time")
          n158 = in-place-cluster #2(w392) -> ("Timing.Started?"=w399:bool)  [unwired: 5 out]
          n159 = Get Date/Time In Seconds() -> (seconds since 1Jan1904=w395:timestamp)
          n160 = Not(x=w399) -> (.not. x?=w400:bool)
          n161 = To Double Precision Float(number=w395) -> (double precision float=w394:dbl)
          n162 = in-place-cluster #2("Timing.Start Time"=w394, "Timing.Elapsed Time"=w396, "Timing.Previous Time"=w396, "Timing.Started?"=w400, "Timing.Paused"=FALSE, "Timing.Set Time"=3.0) -> (w391:T10)
        }
      }
      frame "Timer Paused" {
        # "Pause timer"
        n163 = in-place "In Place Element Structure" {
          n164 = in-place-cluster #3(w402) -> ("Timing.Elapsed Time"=w406:dbl, "Timing.Started?"=w407:bool, "Timing.Paused"=w409:bool)  [unwired: 2 out]
          n165 = Get Date/Time In Seconds() -> (seconds since 1Jan1904=w405:timestamp)
          n166 = Not(x=w409) -> (.not. x?=w408:bool)
          n167 = To Double Precision Float(number=w405) -> (double precision float=w404:dbl)
          n168 = in-place-cluster #3("Timing.Start Time"=w404, "Timing.Elapsed Time"=w406, "Timing.Previous Time"=w406, "Timing.Started?"=w407, "Timing.Paused"=w408) -> (w401:T10)
        }
      }
      frame "Get Elapsed Time" {
        # "Elapsed time = start time + current time - previous time"
        n169 = Unbundle By Name(w417) -> ("Timing.Start Time"=w421:dbl, "Timing.Previous Time"=w419:dbl, "Timing.Paused"=w420:bool, "Timing.Set Time"=w413:dbl)
        n170 = case shown="False" w420 {
          tunnel: w421 -> [w436 _]
          tunnel: w419 -> [w435 w440]
          tunnel: [w434 w440] -> w416
          frame False {
            n171 = Get Date/Time In Seconds() -> (seconds since 1Jan1904=w439:timestamp)
            n172 = To Double Precision Float(number=w439) -> (double precision float=w438:dbl)
            n173 = Subtract(x=w438, y=w436) -> (x-y=w437:dbl)
            n174 = Add(x=w437, y=w435) -> (x+y=w434:dbl)
          }
          frame True {
          }
        }
        n175 = Greater?(x=w416, y=w413) -> (0:w415:bool)
        n176 = case shown="True" w415 {
          tunnel: w414 -> [w425 w430]
          tunnel: w413 -> [_ _]
          tunnel: [w424 w431] -> w412
          tunnel: [TRUE FALSE] -> w411
          tunnel: [FALSE FALSE] -> w410
          frame False {
            n177 = call "Queue Driver_Sender.vi"("Array of States"=cluster{"State":string, "Data":variant}[] [{"State"="Update FP", "Data"=variant}], "Error In"=w425, "Operation"=Queue_Operation_Sender."Enqueue") -> ("Error Out"=w424:errorcluster)  [unwired: 11 in, 1 out]
          }
          frame True {
            n178 = call "Queue Driver_Sender.vi"("Array of States"=cluster{"State":string, "Data":variant}[] [{"State"="Start Timer", "Data"=variant}, {"State"="Update FP", "Data"=variant}], "Error In"=w430, "Operation"=Queue_Operation_Sender."Enqueue") -> ("Error Out"=w431:errorcluster)  [unwired: 11 in, 1 out]
          }
        }
        n179 = Bundle By Name(cluster=w417, "Timing.Elapsed Time"=w416, "Status indicators.Data Sent"=w411, "Status indicators.Receiver Offline"=w410) -> (w418:T10)
      }
      frame "***Error***" {
      }
      frame "Consumer Error" {
        # "Handle the Consumer errors if occured"
        n180 = Unbundle By Name(w444) -> ("State"=w443:string)
        n181 = Unbundle By Name(w446) -> ("code"=w453:i32, "source"=w452:string)
        n182 = call <vilib>:"Clear Errors.vi"("error in (no error)"=w446, "specific error code to clear (0: all)"=w453) -> ("error out"=w455:errorcluster)  [unwired: 4 in, 1 out]
        n183 = Format Into String(format string="CONSUMER ERROR\nError occurred in state \"%s\"!!\nError Code: %d\nError Source: %s\n\nDo you wish to continue?", error in=w455, w443, w453, w452) -> (resulting string=w451:string, error out=w447:errorcluster)  [unwired: 1 in]
        n184 = Two Button Dialog(message=w451, 1:"Exit" ("F button name (\"Cancel\")"), 2:"Continue" ("T button name (\"OK\")")) -> (T button?=w448:bool)
        n185 = case "Continue?" shown="True" w448 {
          tunnel: w447 -> [w459 w465]
          tunnel: [w458 w462] -> w445
          frame False {
            # "Exit"
            n186 = call "Queue Driver_Sender.vi"("Array of States"=cluster{"State":string, "Data":variant}[] [{"State"="Exit", "Data"=variant}], "Error In"=w459, "Operation"=Queue_Operation_Sender."Enqueue") -> ("Error Out"=w458:errorcluster)  [unwired: 11 in, 1 out]
          }
          frame True {
            # "Continue"
            n187 = call "Queue Driver_Sender.vi"("Error In"=w465, "Operation"=Queue_Operation_Sender."Flush") -> ("Error Out"=w463:errorcluster)  [unwired: 12 in, 1 out]
            n188 = call "Queue Driver_Sender.vi"("Array of States"=cluster{"State":string, "Data":variant}[] [{"State"="Initialize", "Data"=variant}, {"State"="Enable Disable Controls", "Data"=variant}, {"State"="Update FP", "Data"=variant}], "Error In"=w463, "Operation"=Queue_Operation_Sender."Enqueue") -> ("Error Out"=w462:errorcluster)  [unwired: 11 in, 1 out]
          }
        }
      }
      frame "Producer Error" {
        # "Handle the Producer errors if occured"
        n189 = Variant To Data(error in=w471, type=errorcluster {"status"=FALSE, "code"=0, "source"=""} ("error IO"), Variant=w473) -> (data=w469:errorcluster, error out=w472:errorcluster)
        n190 = Unbundle By Name(w469) -> ("code"=w468:i32, "source"=w467:string)
        n191 = Format Into String(format string="PRODUCER ERROR\nError occurred..!!\nError Code: %d\nError Source: %s\n\nDo you wish to continue?", error in=w472, w468, w467) -> (resulting string=w479:string, error out=w475:errorcluster)  [unwired: 1 in]
        n192 = Two Button Dialog(message=w479, 1:"Exit" ("F button name (\"Cancel\")"), 2:"Continue" ("T button name (\"OK\")")) -> (T button?=w476:bool)
        n193 = case "Continue?" shown="True" w476 {
          tunnel: w475 -> [w483 w490]
          tunnel: [w482 w487] -> w474
          frame False {
            # "Exit"
            n194 = call "Queue Driver_Sender.vi"("Array of States"=cluster{"State":string, "Data":variant}[] [{"State"="Exit", "Data"=variant}], "Error In"=w483, "Operation"=Queue_Operation_Sender."Enqueue") -> ("Error Out"=w482:errorcluster)  [unwired: 11 in, 1 out]
          }
          frame True {
            # "Continue"
            n195 = call "Queue Driver_Sender.vi"("Error In"=w490, "Operation"=Queue_Operation_Sender."Flush") -> ("Error Out"=w488:errorcluster)  [unwired: 12 in, 1 out]
            n196 = call "Queue Driver_Sender.vi"("Array of States"=cluster{"State":string, "Data":variant}[] [{"State"="Initialize", "Data"=variant}, {"State"="Enable Disable Controls", "Data"=variant}, {"State"="Update FP", "Data"=variant}], "Error In"=w488, "Operation"=Queue_Operation_Sender."Enqueue") -> ("Error Out"=w487:errorcluster)  [unwired: 11 in, 1 out]
          }
        }
      }
      frame "***Exit***" {
      }
      frame "Exit" {
        # "Exit the state machine"
        n197 = call "Queue Driver_Sender.vi"("Error In"=w498, "Operation"=Queue_Operation_Sender."Flush") -> ("Error Out"=w499:errorcluster)  [unwired: 12 in, 1 out]
        n198 = call "Queue Driver_Sender.vi"("Error In"=w499, "Operation"=Queue_Operation_Sender."Release") -> ("Error Out"=w496:errorcluster)  [unwired: 12 in, 1 out]
        n199 = call "User_Event_LV2.vi"("STOP"=T17 {"STOP"=TRUE}, "Error In"=w496, "Operation"=User_Event_Operation."Generate") -> ("Error Out"=w495:errorcluster)  [unwired: 11 in, 1 out]
      }
    }
  }
  n200 = call "User_Event_LV2.vi"("Error In"=w16, "Operation"=User_Event_Operation."Destroy") -> ("Error Out"=w15:errorcluster)  [unwired: 12 in, 1 out]
  n201 = Unregister For Events(event registration refnum=w13, error in=w15) -> (error out=w14:errorcluster)
  n202 = Merge Errors(w14, w26) -> (w2:errorcluster)
  n203 = disable-structure shown="RUN_TIME_ENGINE==True" {
    disable-tunnel: w2 -> [w504 w506]
    disable-tunnel: [w504 w505] -> w1
    frame condition #0 (active) {
    }
    frame condition #1 {
      n204 = control-ref of="This VI"() -> (w507:refnum<vi>)
      n205 = invoke class="VI" method="FP.Close"(reference=w507, error in=w506) -> (error out=w505:errorcluster)  [unwired: 1 in, 2 out]
    }
  }
  "error out" <- w1
